vi "Write Instrument Info Array.vi"(8 "error in (no error)":errorcluster, 10 "Instrument Info Array":T1[](array[typedef]), 11 "Power Meter Base in":refnum<class "Power Meter Base.lvclass">) -> (0 "error out":errorcluster, 3 "Power Meter Base out":refnum<class "Power Meter Base.lvclass">)   [LabVIEW 2023, in "RFFixtureCharact.Instruments.lvlib" / "Power Meter Base.lvclass"]
uses:
  Power Meter Base.lvclass
  Type Definitions/Instrument Info.ctl
  Power Meter Base.lvclass/Power Meter Base.ctl
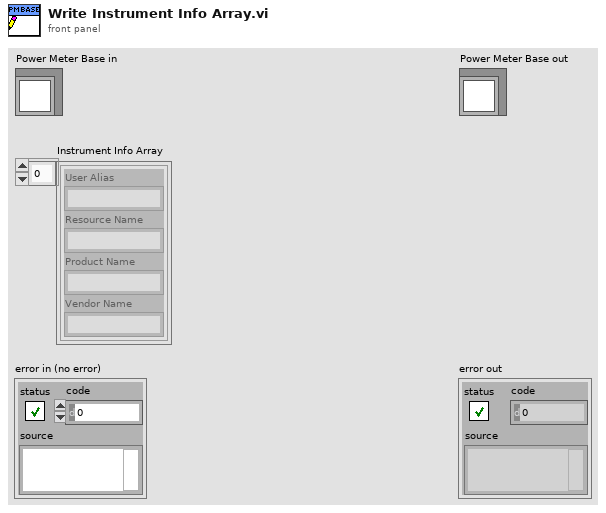
[diagram p1: front panel]
types:
  T1 = typedef "RFFixtureCharact.Instruments.lvlib/Power Meter Base.lvclass/Instrument Info.ctl" = cluster{"User Alias":string, "Resource Name":string, "Product Name":string, "Vendor Name":string}
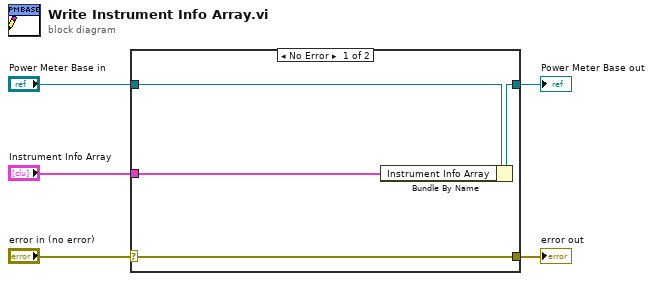
[diagram p0: block diagram]
diagram:
  n1 = case shown="No Error" "error in (no error)" {
    selector: "error in (no error)" -> [w9 w10]
    tunnel: [w9 w10] -> w4
    tunnel: [w7 w11] -> w2
    tunnel: "Power Meter Base in" -> [w8 w11]
    tunnel: "Instrument Info Array" -> [w6 _]
    frame No Error {
      n2 = Bundle By Name(cluster=w8, "Instrument Info Array"=w6) -> (w7:refnum<class "Power Meter Base.lvclass">)
    }
    frame Error {
    }
  }
  "error out" <- w4
  "Power Meter Base out" <- w2
